vi "VIForDiff.vi"() -> ()   [LabVIEW 2015]
panel:
  out "zy":dbl
  in  "x":dbl
  in  "y":dbl
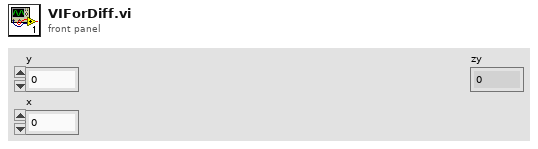
[diagram p1: front panel]
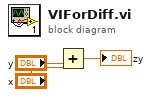
[diagram p0: block diagram]
diagram:
  n1 = Add(x="x", y="y") -> (x+y=→"zy":dbl)
